vi "AlliGator Get Parameter Map Data.vi"(0 "Multiple Parameters":dbl[][](array[numeric]), 1 "Compute Parameter Map":bool, 3 "Output ROI centers?":bool, 5 "X Resolution":i32, 7 "Y Resolution":i32, 11 "Error In":errorcluster, 12 "Map index":i32) -> (4 "Map Data (V x H)":dbl[][](array[numeric]), 6 "Max":dbl, 8 "Min":dbl, 10 "ROI Centers":cluster{"X":dbl, "Y":dbl}[](array[cluster]), 14 "New Map Selected?":bool, 15 "Error Out":errorcluster)   [LabVIEW 2021, in "AlliGator Parameter Map.lvlib"]
doc: "Fills in matrix with fit parameter wherever it has been computed, NaN otherwise."
uses:
  AlliGator Parameter Map.lvlib
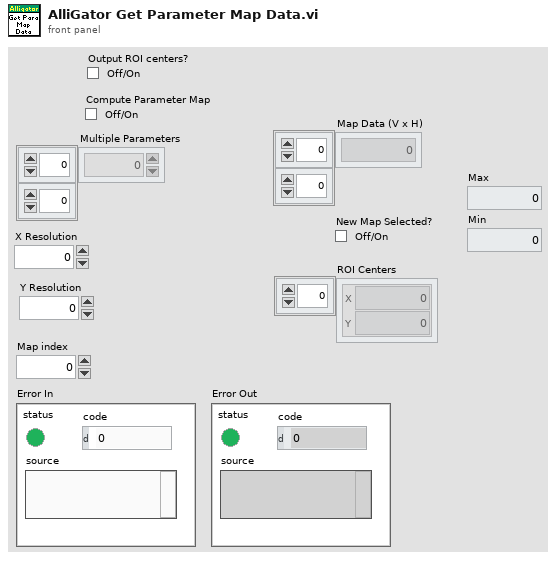
[diagram p1: front panel]
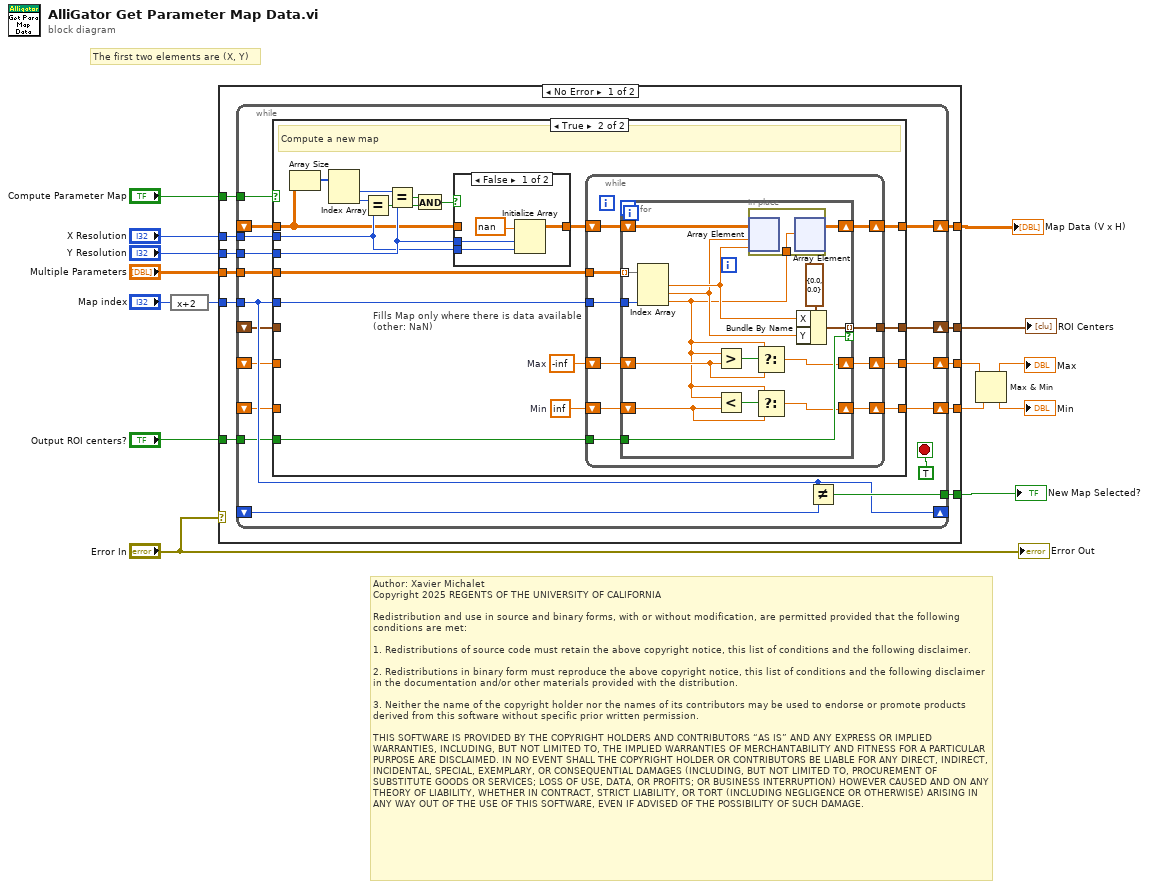
[diagram p0: block diagram]
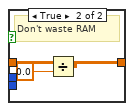
[diagram p3: hidden frame]
diagram:
  # "The first two elements are (X, Y)"
  # "Author: Xavier Michalet\nCopyright 2025 REGENTS OF THE UNIVERSITY OF CALIFORNIA\n\nRedistribution and use in source and binary forms, with or without modification, are permitted provided that the following conditions are met:\n\n1. Redistributions of source code must retain the above copyright notice, this list of conditions and the following disclaimer.\n\n2. Redistributions in binary form must reproduce the above copyright notice, this list of conditions and the following disclaimer in the documentation and/or other materials provided with the distribution.\n\n3. Neither the name of the copyright holder nor the names of its contributors may be used to endorse or promote products derived from this software without specific prior written permission.\n\nTHIS SOFTWARE IS PROVIDED BY THE COPYRIGHT HOLDERS AND CONTRIBUTORS “AS IS” AND ANY EXPRESS OR IMPLIED WARRANTIES, INCLUDING, BUT NOT LIMITED TO, THE IMPLIED WARRANTIES OF MERCHANTABILITY AND FITNESS FOR A PARTICULAR PURPOSE ARE DISCLAIMED. IN NO EVENT SHALL THE COPYRIGHT HOLDER OR CONTRIBUTORS BE LIABLE FOR ANY DIRECT, INDIRECT, INCIDENTAL, SPECIAL, EXEMPLARY, OR CONSEQUENTIAL DAMAGES (INCLUDING, BUT NOT LIMITED TO, PROCUREMENT OF SUBSTITUTE GOODS OR SERVICES; LOSS OF USE, DATA, OR PROFITS; OR BUSINESS INTERRUPTION) HOWEVER CAUSED AND ON ANY THEORY OF LIABILITY, WHETHER IN CONTRACT, STRICT LIABILITY, OR TORT (INCLUDING NEGLIGENCE OR OTHERWISE) ARISING IN ANY WAY OUT OF THE USE OF THIS SOFTWARE, EVEN IF ADVISED OF THE POSSIBILITY OF SUCH DAMAGE."
  n1 = expression code="x+2"("Map index") -> (w5:i32)
  n2 = case shown="No Error" "Error In" {
    tunnel: "Y Resolution" -> [w26 _]
    tunnel: "X Resolution" -> [w25 _]
    tunnel: w5 -> [w24 _]
    tunnel: [w23 _] -> w12
    tunnel: [w22 _] -> w11
    tunnel: "Compute Parameter Map" -> [w21 _]
    tunnel: "Multiple Parameters" -> [w20 _]
    tunnel: [w19 _] -> w7
    tunnel: "Output ROI centers?" -> [w18 _]
    tunnel: [w17 _] -> w4
    tunnel: [w16 _] -> w2
    frame No Error {
      n3 = while {
        tunnel: w20 -> [w42]
        tunnel: w21 -> [w41]
        shift-right: [w43] -> w22
        shift-left: _ -> [w39]
        tunnel: w24 -> [w34]
        shift-right: [w34] -> _
        shift-left: _ -> [w38]
        tunnel: [w37] -> w23
        tunnel: w25 -> [w36]
        tunnel: w26 -> [w35]
        tunnel: w18 -> [w32]
        shift-right: [w33] -> w19
        shift-left: _ -> [w31]
        shift-right: [w30] -> w17
        shift-left: _ -> [w28]
        shift-right: [w29] -> w16
        shift-left: _ -> [w27]
        stop <- TRUE stop-if-true
        n4 = case shown="True" w41 {
          tunnel: [w47 w66] -> w43
          tunnel: w42 -> [_ w65]
          tunnel: w39 -> [w47 w52]
          tunnel: w34 -> [_ w63]
          tunnel: w36 -> [_ w56]
          tunnel: w35 -> [_ w58]
          tunnel: [w46 w62] -> w33
          tunnel: w32 -> [_ w61]
          tunnel: w31 -> [w46 _]
          tunnel: [w45 w49] -> w30
          tunnel: [w44 w48] -> w29
          tunnel: w28 -> [w45 _]
          tunnel: w27 -> [w44 _]
          frame False {
            # "use old map"
          }
          frame True {
            w50 = inf  # Min
            w51 = -inf  # Max
            # "Compute a new map"
            n5 = Array Size(array=w52) -> (size(s)=w60:i32[])
            n6 = Index Array(array=w60) -> (element #1=w59:i32, element #2=w57:i32)  [unwired: 2 in]
            n7 = Equal?(x=w57, y=w56) -> (x = y?=w54:bool)
            n8 = Equal?(x=w59, y=w58) -> (x = y?=w55:bool)
            n9 = And(x=w55, y=w54) -> (x .and. y?=w53:bool)
            n10 = case shown="False" w53 {
              tunnel: [w97 w99] -> w64
              tunnel: w58 -> [w96 _]
              tunnel: w56 -> [w95 _]
              tunnel: w52 -> [_ w101]
              frame False {
                n11 = Initialize Array(nan, w96, w95) -> (w97:dbl[][])
              }
              frame True {
                # "Don't waste RAM"
                n12 = Divide(x=w101, y=0.0) -> (x/y=w99:dbl[][])
              }
            }
            n13 = while "Fills Map only where there is data available (other: NaN)" {
              shift-right: [w77] -> w66
              shift-left: w64 -> [w74]
              tunnel: w65 -> [w75]
              tunnel: w63 -> [w73]
              tunnel: [w72] -> w62
              tunnel: w61 -> [w71]
              shift-right: [w69] -> w49
              shift-left: w51 -> [w70]
              shift-right: [w67] -> w48
              shift-left: w50 -> [w68]
              stop <- TRUE stop-if-true
              n14 = for {
                shift-right: [w92] -> w77
                shift-left: w74 -> [w93]
                tunnel: w75 -> [w91] mode=indexing
                tunnel: w73 -> [w90]
                tunnel: [w86] -> w72 mode=indexing if=w85
                tunnel: w71 -> [w85]
                shift-right: [w82] -> w69
                shift-left: w70 -> [w83]
                shift-right: [w78] -> w67
                shift-left: w68 -> [w79]
                n15 = Index Array(array=w91, index #3=w90) -> (element #1=w88:dbl, element #2=w87:dbl, element #3=w80:dbl)  [unwired: 2 in]
                n16 = Greater?(x=w80, y=w83) -> (0:w84:bool)
                n17 = Less?(x=w80, y=w79) -> (x < y?=w81:bool)
                n18 = in-place {
                  in-place-border: w80 -> [w94]
                  n19 = in-place-array #1(w93, w87, w88) -> ()  [unwired: 1 out]
                  n20 = in-place-array #1(w94) -> (w92:dbl[][])  [unwired: 2 out]
                }
                n21 = Select(t=w80, s=w84, f=w83) -> (s? t:f=w82:dbl)
                n22 = Select(t=w80, s=w81, f=w79) -> (s? t:f=w78:dbl)
                n23 = Bundle By Name(cluster=cluster{"X":dbl, "Y":dbl} {"X"=0.0, "Y"=0.0} ("ROI Centers"), "X"=w88, "Y"=w87) -> (w86:cluster{"X":dbl, "Y":dbl})
              }
            }
          }
        }
        n24 = Not Equal?(x=w34, y=w38) -> (x != y?=w37:bool)
      }
    }
    frame Error {
    }
  }
  "New Map Selected?" <- w12
  "Map Data (V x H)" <- w11
  "ROI Centers" <- w7
  n25 = Max & Min(x=w4, y=w2) -> (max(x,y)=→"Max":dbl, min(x,y)=→"Min":dbl)
  "Error Out" <- "Error In"
